vi "SubscribeByType.vi"(5 "Message Transport Interface":refnum<class "Message Transport Interface.lvclass">, 6 "Subscriber Name":string, 7 "Event":refnum<class "Message Interface.lvclass">, 8 "error in (no error)":errorcluster, 11 "Message Broker Interface in":refnum<class "EDA Message Broker Interface Ref.lvclass">=refnum) -> (0 "error out":errorcluster, 3 "Message Broker Interface out":refnum<class "EDA Message Broker Interface Ref.lvclass">)   [LabVIEW 2016, in "Stream Mediator.lvlib" / "EDA Message Broker Interface Ref.lvclass"]
doc: "--\nCopyright © 2017 Composed SystemsI All rights reserved.\n\nAuthor: Jon McBee <jon.mcbee@composed.io>\n\nThis library is provided \"AS IS\" ,WITHOUT WARRANTIES OR\nCONDITIONS OF ANY KIND, either express or implied.\n\nComposed Systems -- composed.io\n\nStream 0.0.1.1\nJon McBee - Composed Systems\nCopyright (c) 2017, Composed Systems"
uses:
  <userlib>/Composed Systems/Stream/Mediator/Classes/EDA Message Broker Interface Ref/EDA Message Broker Interface Ref.lvclass
  C:/Program Files (x86)/National Instruments/LabVIEW 2016/user.lib/Composed Systems/Stream/Mediator/Classes/Message Broker Interface Ref/Message Broker Interface Ref.lvclass
  <userlib>/Composed Systems/Stream/Mediator/Classes/Message Transport Interface/Message Transport Interface.lvclass
  <userlib>/Composed Systems/Stream/Mediator/Classes/Message Interface/Message Interface.lvclass
  <userlib>/Composed Systems/Stream/Mediator/Classes/Message Broker/Message Broker.lvclass
  <userlib>/Composed Systems/Stream/Mediator/Classes/Message Broker Interface Ref/Message Broker Interface Ref.lvclass
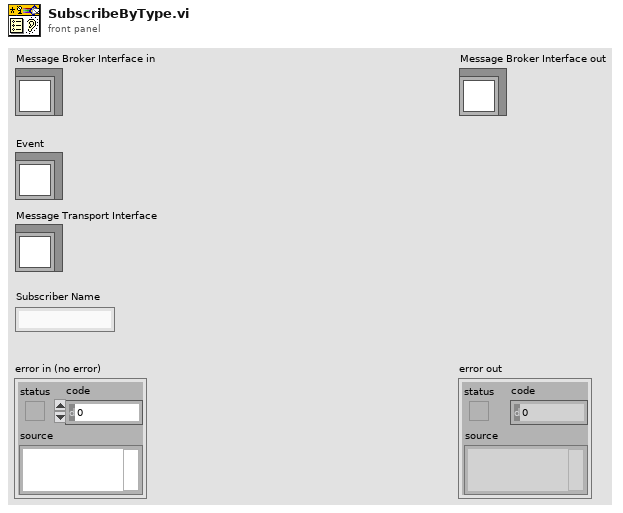
[diagram p1: front panel]
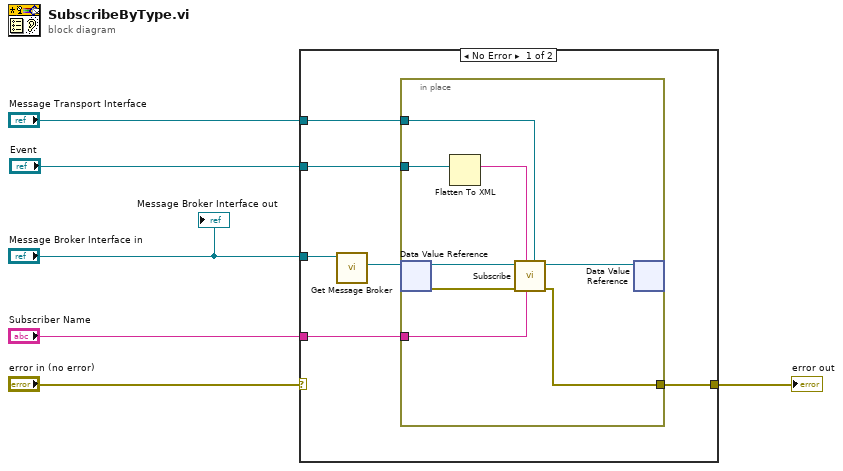
[diagram p0: block diagram]
diagram:
  n1 = case shown="No Error" "error in (no error)" {
    selector: "error in (no error)" -> [_ w21]
    tunnel: [w7 w21] -> w5
    tunnel: "Subscriber Name" -> [w8 _]
    tunnel: "Message Broker Interface in" -> [w12 _]
    tunnel: "Message Transport Interface" -> [w10 _]
    tunnel: "Event" -> [w9 _]
    frame No Error {
      n2 = call <userlib>:"Get Message Broker.vi"("Message Broker Interface Ref in"=w12) -> ("Broker"=w11:refnum<data-value>)  [unwired: 8 in, 2 out]
      n3 = in-place {
        in-place-border: w10 -> [w18]
        in-place-border: w9 -> [w17]
        in-place-border: w8 -> [w15]
        in-place-border: [w13] -> w7
        n4 = in-place-dvr #1(w11) -> (w20:refnum<class "Message Broker.lvclass">, w14:errorcluster)
        n5 = Flatten To XML(anything=w17) -> (xml string=w16:string)
        n6 = call <userlib>:"Subscribe.vi"("Message Transport Interface"=w18, "Subscriber Name"=w15, "Topic Name"=w16, "error in (no error)"=w14, "Message Broker in"=w20) -> ("error out"=w13:errorcluster, "Message Broker out"=w19:refnum<class "Message Broker.lvclass">)  [unwired: 4 in, 1 out]
        n7 = in-place-dvr #1(w19) -> ()  [unwired: 2 out]
      }
    }
    frame Error {
    }
  }
  "error out" <- w5
  "Message Broker Interface out" <- "Message Broker Interface in"
